vi "Preprocess Auto.vi"(9 "Is Blue Alliance?":bool, 10 "Start Time":dbl, 11 "appended path":path) -> (1 "Positions":cluster{"x":dbl, "y":dbl, "th":dbl}[](array[cluster]), 2 "Array":T1(array[cluster]), 3 "Finish Time":dbl, 4 "Velocities":T2[](array[typedef]), 5 "Zero Velocity?":bool[](array[boolean]))   [LabVIEW 2023]
uses:
  swerve/Type Definitions/Data/Robot Velocities.ctl
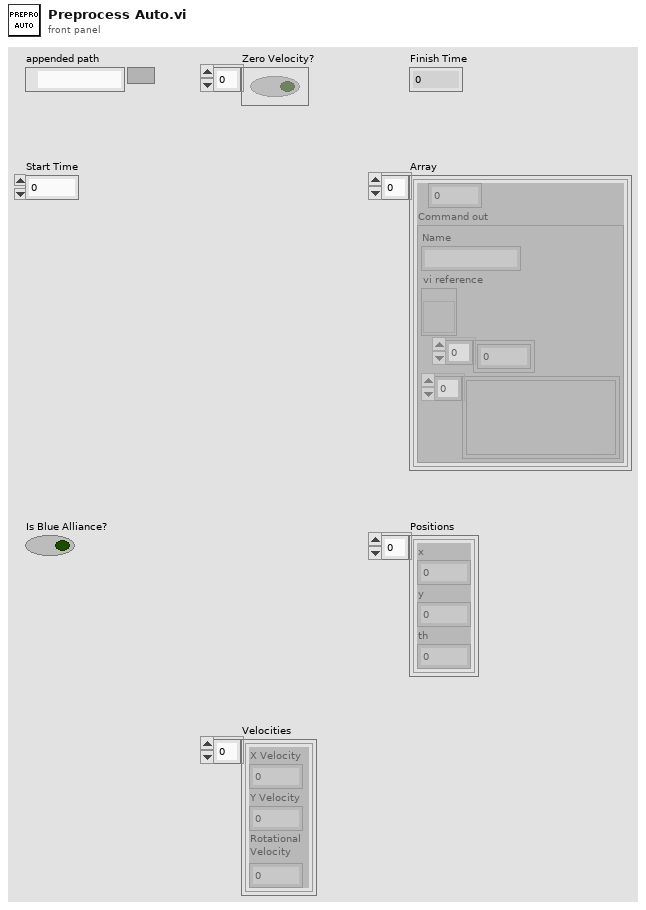
[diagram p1: front panel]
types:
  T1 = cluster{dbl, "Command out":cluster{"Name":string, "vi reference":refnum<vi>, i32[], variant[]}}[]
  T2 = typedef "Robot Velocities.ctl" = cluster{"X Velocity":dbl, "Y Velocity":dbl, "Rotational \nVelocity":dbl}
  T3 = typedef "Single Cmd Info.ctl" = cluster{"Name":string, "CPTM.DataType":variant, "All Control Values Variant":cluster{"Name":string, "Variant Data":variant}[], "icon full":T4, "icon scaled":T4, "Path":path, "Subsystem Color":u32}
  T4 = typedef "imagedata.ctl" = cluster{"image type":i32, "image depth":i32, "image":u8[], "mask":u8[], "colors":u32[], "Rectangle":cluster{"left":i16, "top":i16, "right":i16, "bottom":i16}}
  T5 = cluster{"Name":string, "vi reference":refnum<vi>, i32[], variant[]}
  T6 = cluster{dbl, "Command out":cluster{"Name":string, "vi reference":refnum<vi>, i32[], variant[]}}
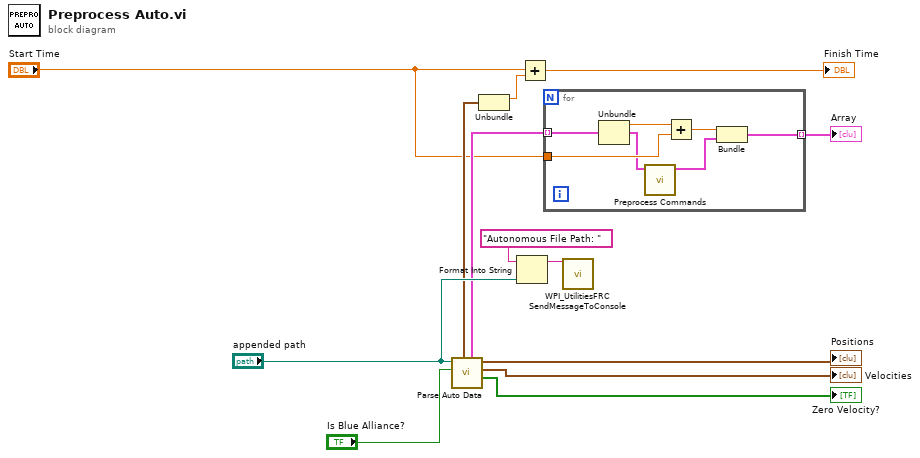
[diagram p0: block diagram]
diagram:
  n1 = call "Parse Auto Data.vi"("Is Blue Alliance?"="Is Blue Alliance?", "path"="appended path") -> ("Zero Velocity?"=→"Zero Velocity?":bool[], "Velocities"=→"Velocities":T2[], "Positions"=→"Positions":cluster{"x":dbl, "y":dbl, "th":dbl}[], "Commands out"=w8:cluster{"Time (s)":dbl, T3, bool}[], "Overall"=w4:cluster{"Time (s)":dbl, "Distance (ft)":dbl})  [unwired: 5 in]
  n2 = Unbundle(w4) -> ("Time (s)"=w13:dbl)  [unwired: 1 out]
  n3 = Format Into String(initial string="Autonomous File Path: ", "appended path") -> (resulting string=w11:string)  [unwired: 2 in, 1 out]
  n4 = Add(x="Start Time", y=w13) -> (x+y=→"Finish Time":dbl)
  n5 = for {
    tunnel: "Start Time" -> [w19]
    tunnel: w8 -> [w18] mode=indexing
    tunnel: [w14] -> w2 mode=indexing
    n6 = Unbundle(w18) -> ("Time (s)"=w20:dbl, w17:T3)  [unwired: 1 out]
    n7 = call "Preprocess Commands.vi"("Command In"=w17) -> ("Command out"=w15:T5)  [unwired: 10 in]
    n8 = Add(x=w20, y=w19) -> (x+y=w16:dbl)
    n9 = Bundle(w16, "Command out"=w15) -> (w14:T6)  [unwired: 1 in]
  }
  "Array" <- w2
  n10 = call <vilib>:"WPI_UtilitiesFRC SendMessageToConsole.vi"("Message"=w11) -> ()  [unwired: 14 in, 1 out]
